vi "Find Serial VISA Names.vi"(1 "Search Mode":T1=2 items=["Canonical Names Only"=0, "Aliases Only"=2, "Include Matching Aliases"=3, "Include All Aliases"=4], 11 "error in":errorcluster) -> (4 "ASRL VISA":string[](array[string]), 8 "resources found":i32, 15 "error out":errorcluster)   [LabVIEW 2017]
uses:
  <vilib>/Instr/_visa.llb/VISA Find Search Mode.ctl
panel:
  out "VISA resources found":string[](array[string])
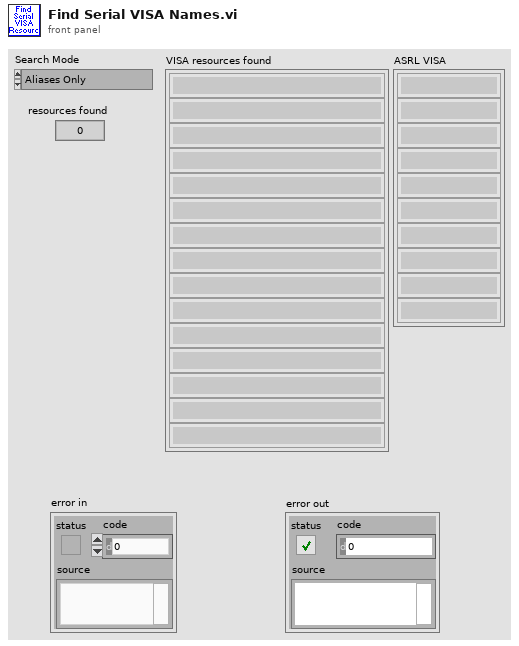
[diagram p1: front panel]
types:
  T1 = typedef "VISA Find Search Mode.ctl" = u32
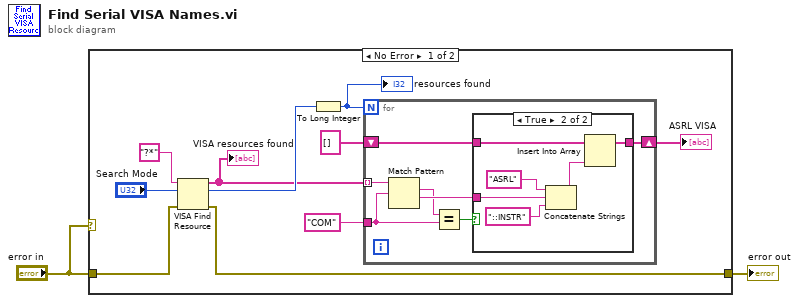
[diagram p0: block diagram]
diagram:
  n1 = case shown="No Error" "error in" {
    tunnel: "error in" -> [w10 w27]
    tunnel: [w3 w27] -> w2
    frame No Error {
      n2 = VISA Find Resource(8:w10, 10:"Search Mode", 11:"?*" ("expression (\"?*\")")) -> (0:w3:errorcluster, 2:w9:u32, 3:w7:string[])
      "VISA resources found" <- w7
      n3 = To Long Integer(number=w9) -> (32bit integer=w8:i32)
      "resources found" <- w8
      n4 = for {
        N: w8 -> [_]
        tunnel: w7 -> [w19] mode=indexing
        tunnel: "COM" ("regular expression") -> [w16]
        shift-right: [w13] -> w4
        shift-left: string[] [] -> [w14]
        n5 = Match Pattern(string=w19, regular expression=w16) -> (match substring=w15:string, after substring=w17:string)  [unwired: 1 in, 2 out]
        n6 = Equal?(x=w15, y=w16) -> (x = y?=w18:bool)
        n7 = case shown="True" w18 {
          tunnel: w17 -> [_ w25]
          tunnel: [w20 w21] -> w13
          tunnel: w14 -> [w20 w22]
          frame False {
          }
          frame True {
            n8 = Concatenate Strings("ASRL", w25, "::INSTR") -> (w23:string)
            n9 = Insert Into Array(array=w22, new element=w23) -> (w21:string[])  [unwired: 1 in]
          }
        }
      }
      "ASRL VISA" <- w4
    }
    frame Error {
    }
  }
  "error out" <- w2
